vi "Solenoid Activate.vi"(9 "Reverse is On":bool, 10 "Input Boolean":bool, 11 "Solenoid Name":string="GearHopper") -> ()   [LabVIEW 2016]
uses:
  <vilib>/Rock Robotics/WPI/Solenoid/WPI_SolenoidValue.ctl
  <vilib>/Rock Robotics/WPI/Solenoid/WPI_SolenoidSetEnum.vi
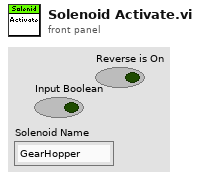
[diagram p1: front panel]
types:
  T1 = typedef "WPI_SolenoidValue.ctl" = enum16{"Off", "On", "Forward", "Reverse"}
  T2 = typedef "WPI_SolenoidDevRef.ctl" = cluster{"DevStatus":errorcluster, "Pneumatics Control Module":u8, "Forward Solenoid Channel":T3, "Reverse Solenoid Channel":T3}
  T3 = typedef "WPI_SolenoidChannel.ctl" = enum8{"Solenoid 0", "Solenoid 1", "Solenoid 2", "Solenoid 3", "Solenoid 4", "Solenoid 5", "Solenoid 6", "Solenoid 7", "Invalid"}
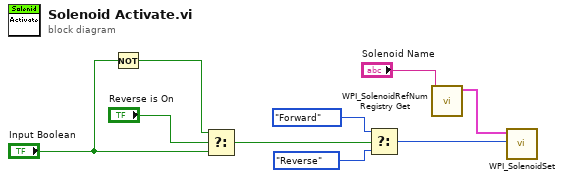
[diagram p0: block diagram]
diagram:
  n1 = Not(x="Input Boolean") -> (.not. x?=w1:bool)
  n2 = Select(t=w1, s="Reverse is On", f="Input Boolean") -> (s? t:f=w4:bool)
  n3 = Select(t=WPI_SolenoidValue."Forward" ("Value"), s=w4, f=WPI_SolenoidValue."Reverse" ("Value")) -> (s? t:f=w9:T1)
  n4 = call <vilib>:"WPI_SolenoidRefNum Registry Get.vi"("refnum name"="Solenoid Name") -> ("SolenoidDevRef"=w6:T2)  [unwired: 9 in, 1 out]
  n5 = call-poly <vilib>:"WPI_SolenoidSet.vi"("Value"=w9, "SolenoidDevRef"=w6) -> ()  [unwired: 8 in, 2 out]
